vi "Collapse Cluster.vi"(8 "error in (no error)":errorcluster, 11 "Framework Configuration in":refnum<class "Framework Configuration.lvclass">) -> (0 "error out":errorcluster, 3 "Framework Configuration out":refnum<class "Framework Configuration.lvclass">)   [LabVIEW 2017, in "DSF Core.lvlib" / "Framework Configuration.lvclass"]
uses:
  Framework Configuration.lvclass
  Framework Configuration.lvclass/Framework Configuration.ctl
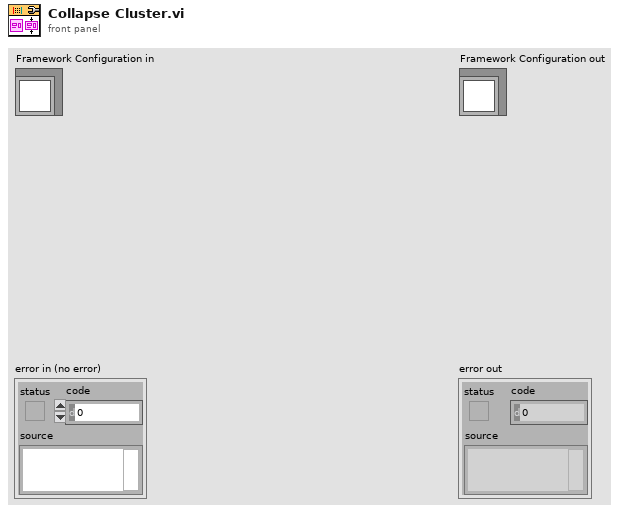
[diagram p1: front panel]
types:
  T1 = typedef "DSF Core.lvlib/DSF Engine Framework Configuration.ctl" = cluster{"Plugins":T2[]}
  T2 = typedef "DSF Core.lvlib/DSF Engine Plugin Configuration.ctl" = cluster{"name":string, "class":string, "cycle timing":T3, "Transfer Groups":T4[], "settings":T10}
  T3 = typedef "DSF Core.lvlib/DSF Timing Info.ctl" = cluster{"priority":u64, "decimation":u64, "offset":u64}
  T4 = typedef "DSF Core.lvlib/DSF Engine Transfer Group Configuration.ctl" = cluster{"name":string, "direction":T5, "cycle timing":T3, "Transfers":T6[], "settings":T10}
  T5 = typedef "DSF Core.lvlib/DSF Direction.ctl" = enum8{"Tx", "Rx"}
  T6 = typedef "DSF Core.lvlib/DSF Engine Transfer Configuration.ctl" = cluster{"name":string, "byte order":T7, "channel configurations":T8[], "settings":T10}
  T7 = typedef "DSF Core.lvlib/DSF Byte Order.ctl" = enum8{"big-endian", "little-endian"}
  T8 = typedef "DSF Core.lvlib/DSF Engine Channel Configuration.ctl" = cluster{"engine offset":u64, "name":string, "data type":T9, "count":u64, "buffer offset":u64, "settings":T10}
  T9 = typedef "DSF Core.lvlib/DSF Data Type.ctl" = enum8{"Bool", "SGL", "DBL", "I8", "I16", "I32", "I64", "U8", "U16", "U32", "U64"}
  T10 = typedef "DSF Core.lvlib/DSF Settings Info.ctl" = cluster{"key":string, "value":string}[]
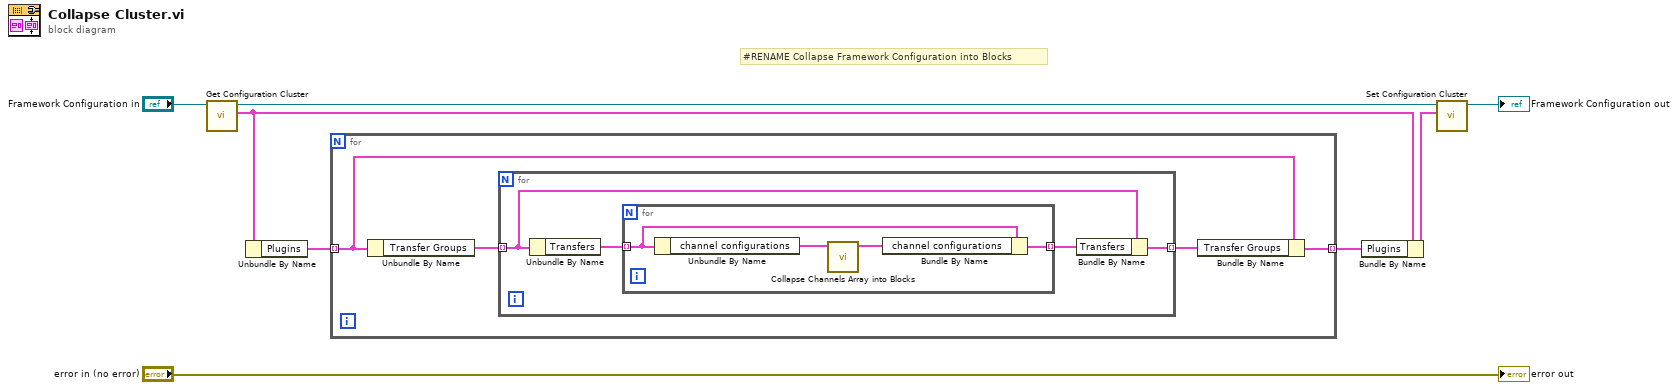
[diagram p0: block diagram]
diagram:
  # "#RENAME Collapse Framework Configuration into Blocks"
  n1 = call "Get Configuration Cluster.vi"("Framework Configuration in"="Framework Configuration in") -> ("Framework Configuration"=w5:T1, "Framework Configuration out"=w7:refnum<class "Framework Configuration.lvclass">)  [unwired: 9 in]
  n2 = Unbundle By Name(w5) -> ("Plugins"=w4:T2[])
  n3 = for {
    tunnel: w4 -> [w11] mode=indexing
    tunnel: [w9] -> w3 mode=indexing
    n4 = Unbundle By Name(w11) -> ("Transfer Groups"=w12:T4[])
    n5 = for {
      tunnel: w12 -> [w15] mode=indexing
      tunnel: [w13] -> w10 mode=indexing
      n6 = Unbundle By Name(w15) -> ("Transfers"=w16:T6[])
      n7 = for {
        tunnel: w16 -> [w19] mode=indexing
        tunnel: [w17] -> w14 mode=indexing
        n8 = Unbundle By Name(w19) -> ("channel configurations"=w20:T8[])
        n9 = call "Collapse Channels Array into Blocks.vi"("channel configurations in"=w20) -> ("channel configurations out"=w18:T8[])  [unwired: 10 in]
        n10 = Bundle By Name(cluster=w19, "channel configurations"=w18) -> (w17:T6)
      }
      n11 = Bundle By Name(cluster=w15, "Transfers"=w14) -> (w13:T4)
    }
    n12 = Bundle By Name(cluster=w11, "Transfer Groups"=w10) -> (w9:T2)
  }
  n13 = Bundle By Name(cluster=w5, "Plugins"=w3) -> (w2:T1)
  n14 = call "Set Configuration Cluster.vi"("Framework Configuration"=w2, "Framework Configuration in"=w7) -> ("Framework Configuration out"=→"Framework Configuration out":refnum<class "Framework Configuration.lvclass">)  [unwired: 9 in]
  "error out" <- "error in (no error)"
